vi "Theta Ref Saturate.vi"(8 "error in (no error)":errorcluster, 11 "Filtered x":dbl) -> (0 "error out":errorcluster, 3 "Theta Ref (Saturated)":sgl)   [LabVIEW 2014]
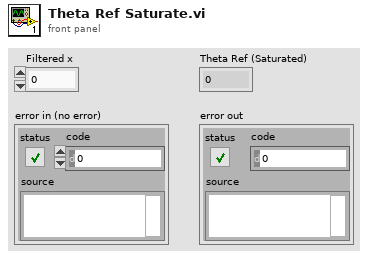
[diagram p1: front panel]
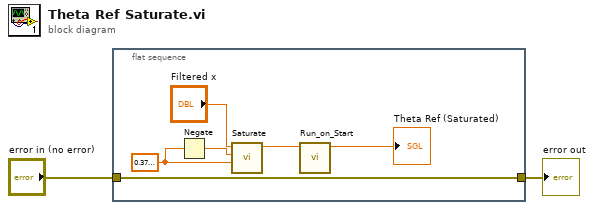
[diagram p0: block diagram]
diagram:
  n1 = flat-sequence {
    tunnel: "error in (no error)" -> [w3]
    tunnel: [w3] -> w1
    frame #0 {
      w4 = sgl 0.37 ("max")
      n2 = Negate(x=w4) -> (-x=w5:sgl)
      n3 = call "Saturate.vi"("Max"=w4, "Min"=w5, "X in"="Filtered x") -> ("X out"=w7:dbl)  [unwired: 8 in]
      n4 = call "Run_on_Start.vi"("val in"=w7) -> ("Val out"=→"Theta Ref (Saturated)":sgl)  [unwired: 10 in]
    }
  }
  "error out" <- w1
